vi "Create Footer Text.vi"(0 "Module Init Timestamp":timestamp, 1 "Module Close Timestamp":timestamp, 2 "Error_Log_Setting":T1, 3 "Total no. of errors reported":i32, 4 "Total no. of errors handled":i32) -> (5 "Footer to be written to error log file":string, 6 "Number of characters":i32)   [LabVIEW 2016, in "Error Manager.lvlib" / "Error Log.lvclass"]
uses:
  Error Log.lvclass
  Error Manager.lvlib
  Settings/Error_Log_Setting (enum).ctl
  Settings/Settings.lvclass
panel:
  # "Input\nInputs to the VI"
  # "Development\nControls or indicators that are useful for development or testing, but which are not outputs of the VI."
  # "Output\nOutputs of the VI"
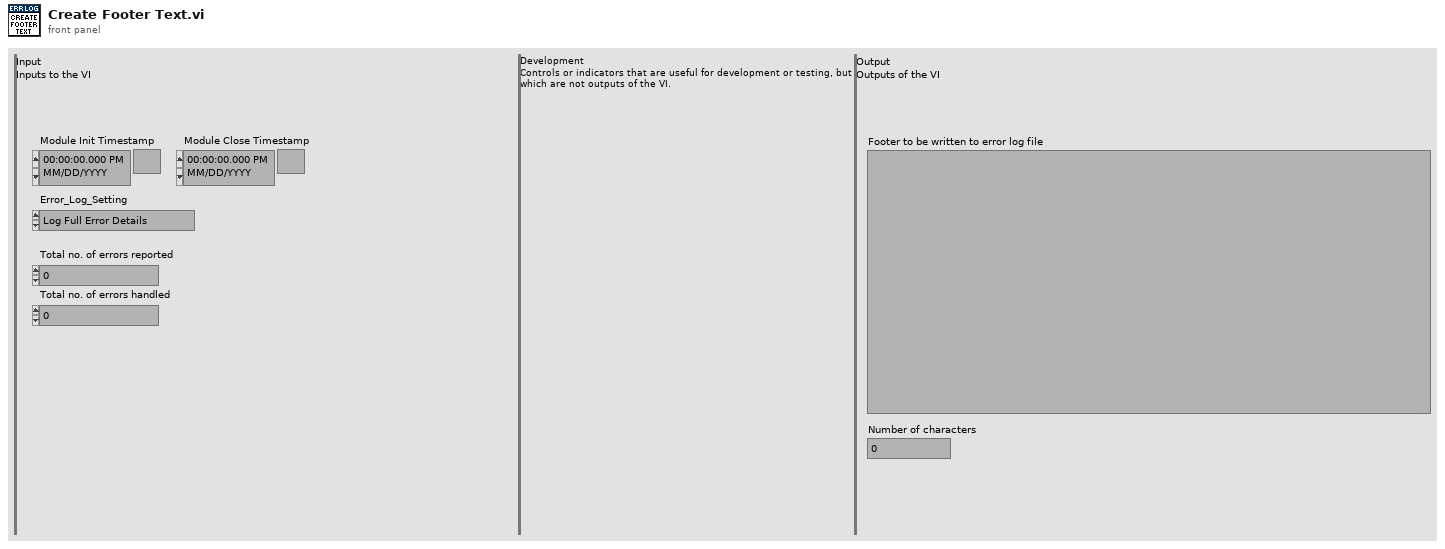
[diagram p1: front panel]
types:
  T1 = typedef "Error Manager.lvlib/Settings.lvclass/Error_Log_Setting (enum).ctl" = enum16{"Log Full Error Details", "Log Error Codes Only", "Do Not Log"}
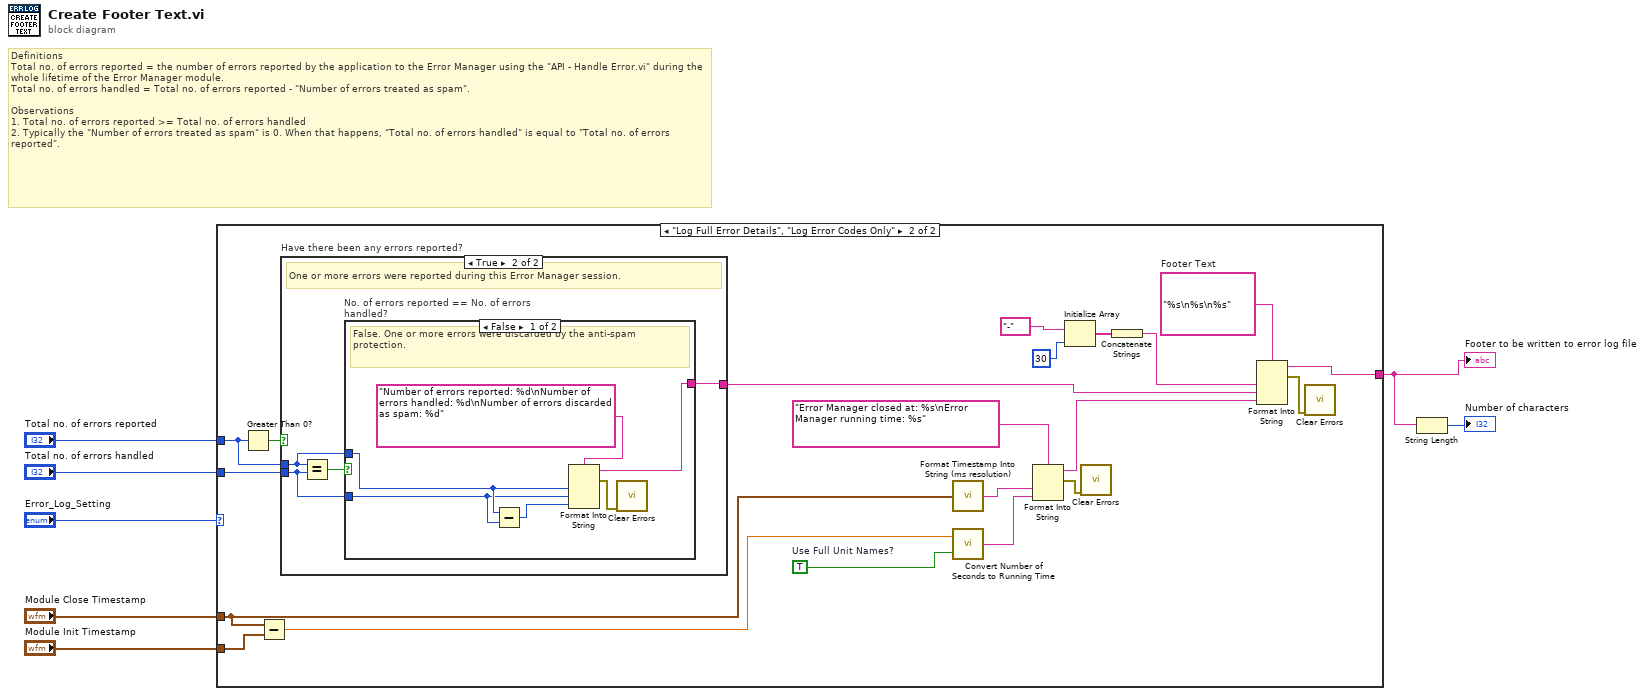
[diagram p0: block diagram]
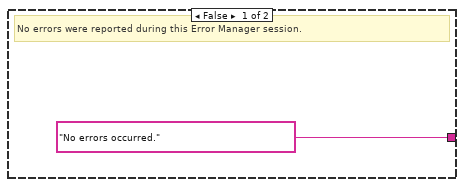
[diagram p3: hidden frame]
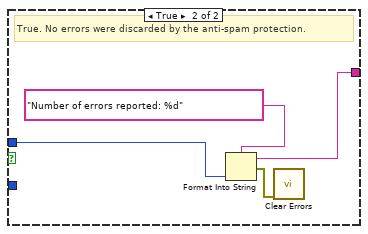
[diagram p4: hidden frame]
diagram:
  # "Definitions\nTotal no. of errors reported = the number of errors reported by the application to the Error Manager using the \"API - Handle Error.vi\" during the whole lifetime of the Error Manager module.\nTotal no. of errors handled = Total no. of errors reported - \"Number of errors treated as spam\".\n\nObservations\n1. Total no. of errors reported >= Total no. of errors handled\n2. Typically the \"Number of errors treated as spam\" is 0. When that happens, \"Total no. of errors handled\" is equal to \"Total no. of errors reported\"."
  n1 = case shown="\"Log Full Error Details\", \"Log Error Codes Only\"" "Error_Log_Setting" {
    tunnel: [_ w23] -> w7
    tunnel: "Total no. of errors reported" -> [_ w15]
    tunnel: "Total no. of errors handled" -> [_ w14]
    tunnel: "Module Close Timestamp" -> [_ w8]
    tunnel: "Module Init Timestamp" -> [_ w20]
    frame "Do Not Log" {
    }
    frame "Log Full Error Details", "Log Error Codes Only" {
      w18 = TRUE  # Use Full Unit Names?
      w25 = "%s\n%s\n%s"  # Footer Text
      n2 = Greater Than 0?(x=w15) -> (x > 0?=w22:bool)
      n3 = Subtract(x=w8, y=w20) -> (x-y=w19:dbl)
      n4 = case "Have there been any errors reported?" shown="True" w22 {
        tunnel: ["No errors occurred." w30] -> w21
        tunnel: w15 -> [_ w31]
        tunnel: w14 -> [_ w29]
        frame False {
          # "No errors were reported during this Error Manager session."
        }
        frame True {
          # "One or more errors were reported during this Error Manager session."
          n5 = Equal?(x=w31, y=w29) -> (x = y?=w32:bool)
          n6 = case "No. of errors reported == No. of errors handled?" shown="False" w32 {
            tunnel: w31 -> [w36 w41]
            tunnel: [w37 w40] -> w30
            tunnel: w29 -> [w35 _]
            frame False {
              # "False. One or more errors were discarded by the anti-spam protection."
              n7 = Subtract(x=w36, y=w35) -> (x-y=w34:i32)
              n8 = Format Into String(format string="Number of errors reported: %d\nNumber of errors handled: %d\nNumber of errors discarded as spam: %d", w36, w35, w34) -> (resulting string=w37:string, error out=w38:errorcluster)  [unwired: 2 in]
              n9 = call <vilib>:"Clear Errors.vi"("error in (no error)"=w38) -> ()  [unwired: 5 in, 2 out]
            }
            frame True {
              # "True. No errors were discarded by the anti-spam protection."
              n10 = Format Into String(format string="Number of errors reported: %d", w41) -> (resulting string=w40:string, error out=w42:errorcluster)  [unwired: 2 in]
              n11 = call <vilib>:"Clear Errors.vi"("error in (no error)"=w42) -> ()  [unwired: 5 in, 2 out]
            }
          }
        }
      }
      n12 = call "Format Timestamp Into String (ms resolution).vi"("Timestamp"=w8) -> ("Timestamp String (ms resolution)"=w27:string)
      n13 = call "Convert Number of Seconds to Running Time.vi"("Use Full Unit Names? (F)"=w18, "Number of seconds elapsed"=w19) -> ("Running Time String"=w17:string)
      n14 = Format Into String(format string="Error Manager closed at: %s\nError Manager running time: %s", w27, w17) -> (resulting string=w16:string, error out=w26:errorcluster)  [unwired: 2 in]
      n15 = Initialize Array("-", 30 ("dimension size")) -> (w10:string[])
      n16 = call <vilib>:"Clear Errors.vi"("error in (no error)"=w26) -> ()  [unwired: 5 in, 2 out]
      n17 = Concatenate Strings(w10) -> (w9:string)
      n18 = Format Into String(format string=w25, w9, w21, w16) -> (resulting string=w23:string, error out=w24:errorcluster)  [unwired: 2 in]
      n19 = call <vilib>:"Clear Errors.vi"("error in (no error)"=w24) -> ()  [unwired: 5 in, 2 out]
    }
  }
  "Footer to be written to error log file" <- w7
  n20 = String Length(string=w7) -> (length=→"Number of characters":i32)
